vi "Read log thresholds.vi"(8 "error in (no error)":errorcluster, 11 "Manage File Request in":refnum<class "Manage File Request.lvclass">) -> (0 "error out":errorcluster, 2 "log thresholds":T1, 3 "Manage File Request out":refnum<class "Manage File Request.lvclass">)   [LabVIEW 2020, in "AIM ARINC 664 Engine.lvlib" / "Implementation.lvlib" / "Frame Logging.lvlib" / "Manage File Request.lvclass"]
uses:
  Manage File Request.lvclass
  Manage File Request.lvclass/Manage File Request.ctl
  Shared/FileSegmentType.ctl
  Monitor Execution Unit/loggingThreshold_types.ctl
  Monitor Execution Unit/Monitor Execution Unit.lvclass
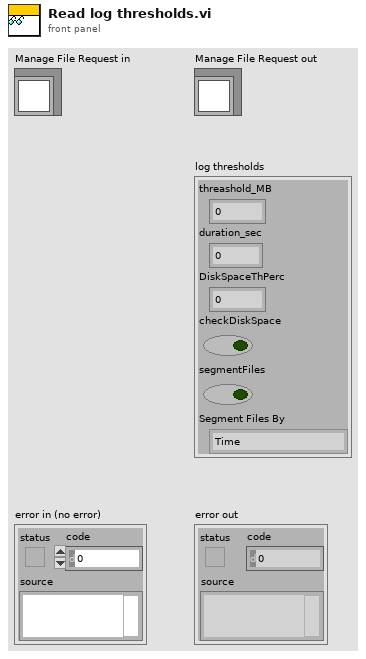
[diagram p1: front panel]
types:
  T1 = typedef "AIM ARINC 664 Engine.lvlib/Implementation.lvlib/Monitor Execution Unit.lvclass/loggingThreshold_types.ctl" = cluster{"threashold_MB":dbl, "duration_sec":dbl, "DiskSpaceThPerc":dbl, "checkDiskSpace":bool, "segmentFiles":bool, "Segment Files By":T2}
  T2 = typedef "FileSegmentType.ctl" = enum16{"Time", "Size"}
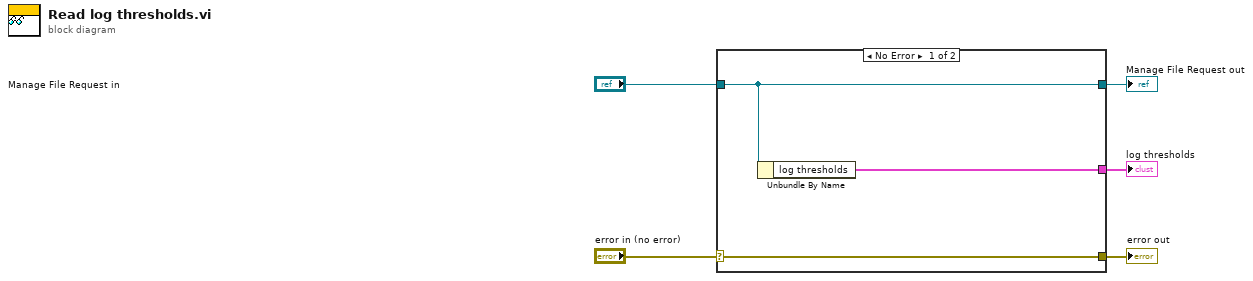
[diagram p0: block diagram]
diagram:
  n1 = case shown="No Error" "error in (no error)" {
    selector: "error in (no error)" -> [w8 w9]
    tunnel: [w8 w9] -> w4
    tunnel: [w7 w10] -> w2
    tunnel: "Manage File Request in" -> [w7 w10]
    tunnel: [w6 _] -> w1
    frame No Error {
      n2 = Unbundle By Name(w7) -> ("log thresholds"=w6:T1)
    }
    frame Error {
    }
  }
  "error out" <- w4
  "Manage File Request out" <- w2
  "log thresholds" <- w1
